vi "Lockin_sensitivity.vi"   [LabVIEW 2019]
uses:
  Instrument_Setup.vi
  Global/Global Variables/global.vi
  Global/Global Variables/Data_Display_global.vi
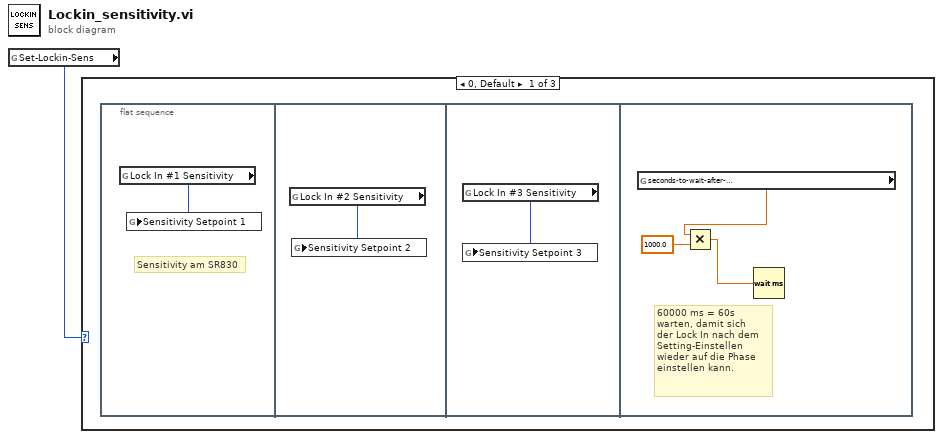
[diagram p0: block diagram]
diagram:
  n1 = global read "Instrument_Setup.vi" "Set-Lockin-Sens"() -> (w1:u16)
  n2 = case shown="0, Default" w1 {
    frame 0, Default {
      n3 = flat-sequence {
        frame #0 {
          # "Sensitivity am SR830"
          n4 = global read "global.vi" "Lock In #1 Sensitivity"() -> (w2:i32)
          n5 = global write "Data_Display_global.vi" "Sensitivity Setpoint 1"(w2) -> ()
        }
        frame #1 {
          n6 = global read "global.vi" "Lock In #2 Sensitivity"() -> (w3:i32)
          n7 = global write "Data_Display_global.vi" "Sensitivity Setpoint 2"(w3) -> ()
        }
        frame #2 {
          n8 = global read "global.vi" "Lock In #3 Sensitivity"() -> (w4:i32)
          n9 = global write "Data_Display_global.vi" "Sensitivity Setpoint 3"(w4) -> ()
        }
        frame #3 {
          # "60000 ms = 60s\nwarten, damit sich\nder Lock In nach dem\nSetting-Einstellen\nwieder auf die Phase\neinstellen kann."
          n10 = global read "Instrument_Setup.vi" "seconds-to-wait-after-\nLock-In-initialization"() -> (w5:dbl)
          n11 = Multiply(x=w5, y=1000.0) -> (x*y=w7:dbl)
          n12 = Wait (ms)(milliseconds to wait=w7) -> ()  [unwired: 1 out]
        }
      }
    }
    frame 1 {
    }
    frame 2 {
    }
  }
